vi "Read Listening HostTypes.vi"(8 "error in (no error)":errorcluster, 11 "Sensor in":refnum<class "Sensor.lvclass">) -> (0 "error out":errorcluster, 2 "Listening HostTypes":T1[](array[typedef]), 3 "Sensor out":refnum<class "Sensor.lvclass">)   [LabVIEW 2012, in "Sensor Definition.lvlib" / "Sensor.lvclass"]
uses:
  Sensor.lvclass
  HostType.ctl
  Sensor.lvclass/Sensor.ctl
  Sensor Definition.lvlib
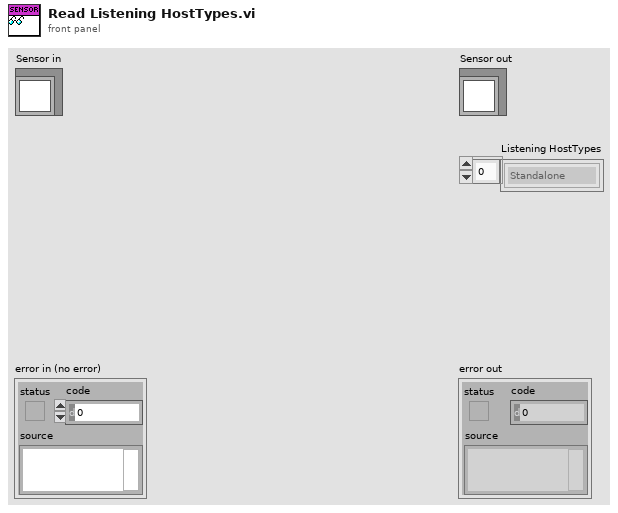
[diagram p1: front panel]
types:
  T1 = typedef "Sensor Definition.lvlib/HostType.ctl" = enum16{"Standalone", "Grid", "MainPane"}
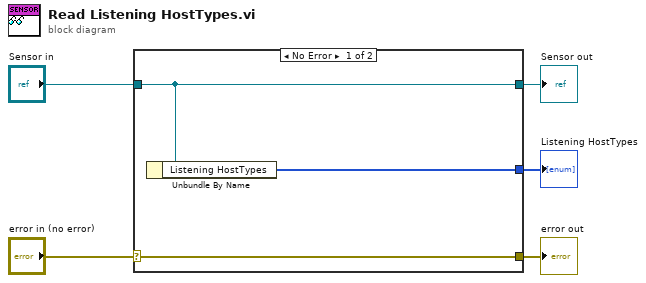
[diagram p0: block diagram]
diagram:
  n1 = case shown="No Error" "error in (no error)" {
    selector: "error in (no error)" -> [w8 w9]
    tunnel: [w8 w9] -> w4
    tunnel: [w7 w10] -> w2
    tunnel: "Sensor in" -> [w7 w10]
    tunnel: [w6 _] -> w1
    frame No Error {
      n2 = Unbundle By Name(w7) -> ("Listening HostTypes"=w6:T1[])
    }
    frame Error {
    }
  }
  "error out" <- w4
  "Sensor out" <- w2
  "Listening HostTypes" <- w1
